vi "Read.vi"(8 "error in":errorcluster, 10 "Channel":string, 11 "Buffer Lossless DBL in":refnum<class "Buffer Lossless DBL.lvclass">) -> (0 "error out":errorcluster, 1 "empty?":bool, 2 "Waveform":waveform(dbl), 3 "Buffer Lossless DBL out":refnum<class "Buffer Lossless DBL.lvclass">)   [LabVIEW 2024, in "Buffer Lossless DBL.lvclass"]
uses:
  Buffer Lossless DBL.lvclass
  Buffer Lossless DBL.lvclass/Buffer Lossless DBL.ctl
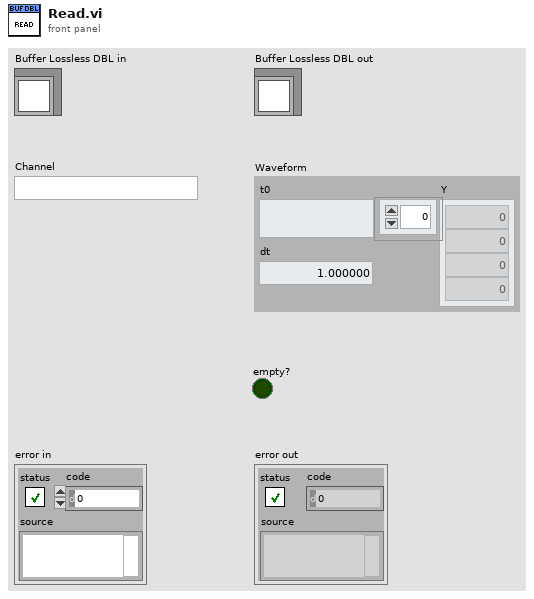
[diagram p1: front panel]
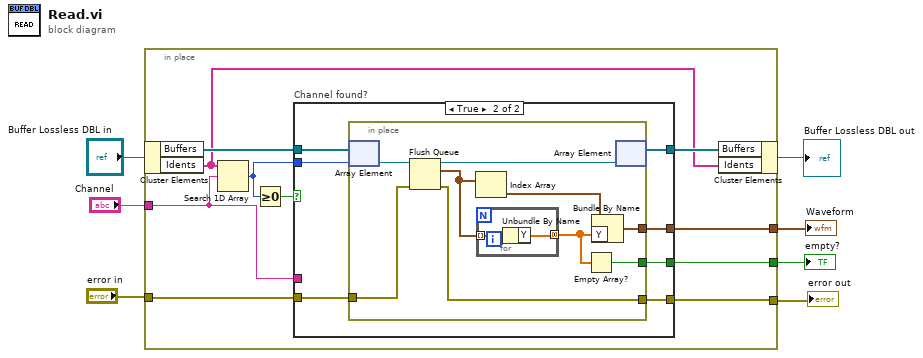
[diagram p0: block diagram]
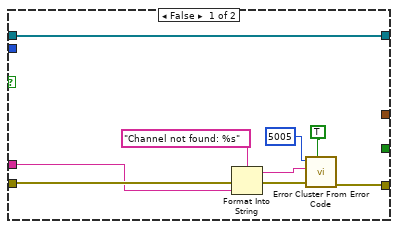
[diagram p2: hidden frame]
diagram:
  n1 = in-place {
    in-place-border: "Channel" -> [w8]
    in-place-border: "error in" -> [w17]
    in-place-border: [w16] -> w2
    in-place-border: [w15] -> w1
    in-place-border: [w9] -> w3
    n2 = in-place-cluster #1("Buffer Lossless DBL in") -> ("Buffers"=w12:refnum<queue>[], "Idents"=w10:string[])
    n3 = Search 1D Array(1D array=w10, element=w8) -> (index of element=w13:i32)  [unwired: 1 in]
    n4 = Greater Or Equal To 0?(x=w13) -> (x >= 0?=w14:bool)
    n5 = case "Channel found?" shown="True" w14 {
      tunnel: w17 -> [w21 w33]
      tunnel: [w20 w31] -> w16
      tunnel: [_ w32] -> w15
      tunnel: w13 -> [_ w29]
      tunnel: w12 -> [w19 w30]
      tunnel: [w19 w28] -> w11
      tunnel: [_ w27] -> w9
      tunnel: w8 -> [w18 _]
      frame False {
        n6 = Format Into String(format string="Channel not found: %s", error in=w21, w18) -> (resulting string=w22:string, error out=w24:errorcluster)  [unwired: 1 in]
        n7 = call <vilib>:"Error Cluster From Error Code.vi"("show call chain? (False)"=TRUE, "error in (no error)"=w24, "error message (\"\")"=w22, "error code (0)"=5005) -> ("error out"=w20:errorcluster)  [unwired: 5 in]
      }
      frame True {
        n8 = in-place {
          in-place-border: w33 -> [w42]
          in-place-border: [w36] -> w32
          in-place-border: [w41] -> w31
          in-place-border: [w34] -> w27
          n9 = in-place-array #2(w30, w29) -> (w40:refnum<queue>)
          n10 = Flush Queue(queue=w40, error in (no error)=w42) -> (queue out=w39:refnum<queue>, remaining elements=w38:waveform(dbl)[], error out=w41:errorcluster)
          n11 = Index Array(array=w38) -> (element=w37:waveform(dbl))  [unwired: 1 in]
          n12 = for {
            tunnel: w38 -> [w44] mode=indexing
            tunnel: [w43] -> w35 mode=concatenating
            n13 = Unbundle By Name(w44) -> ("Y"=w43:dbl[])
          }
          n14 = Empty Array?(array=w35) -> (empty?=w34:bool)
          n15 = Bundle By Name(cluster=w37, "Y"=w35) -> (w36:waveform(dbl))
          n16 = in-place-array #2(w39) -> (w28:refnum<queue>[])  [unwired: 1 out]
        }
      }
    }
    n17 = in-place-cluster #1("Buffers"=w11, "Idents"=w10) -> (→"Buffer Lossless DBL out":refnum<class "Buffer Lossless DBL.lvclass">)
  }
  "error out" <- w2
  "empty?" <- w3
  "Waveform" <- w1
